vi "in_1d interp.vi"(7 "method":i32(ring) items=["nearest", "linear", "spline", "cubic Hermite", "Lagrange"], 9 "xi":dbl[](array[numeric]), 10 "Y":dbl[](array[numeric]), 11 "X":dbl[](array[numeric])) -> (0 "error":i32, 3 "yi":dbl[](array[numeric]))   [LabVIEW 2011, in "NI_Gmath.lvlib"]
uses:
  NI_Gmath.lvlib
  NI_AALPro.lvlib
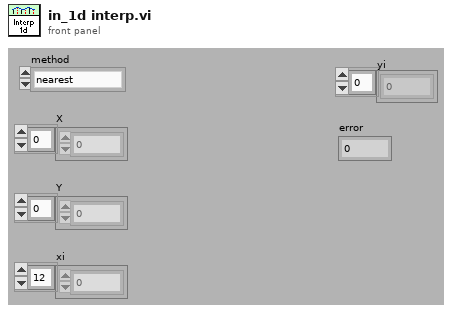
[diagram p1: front panel]
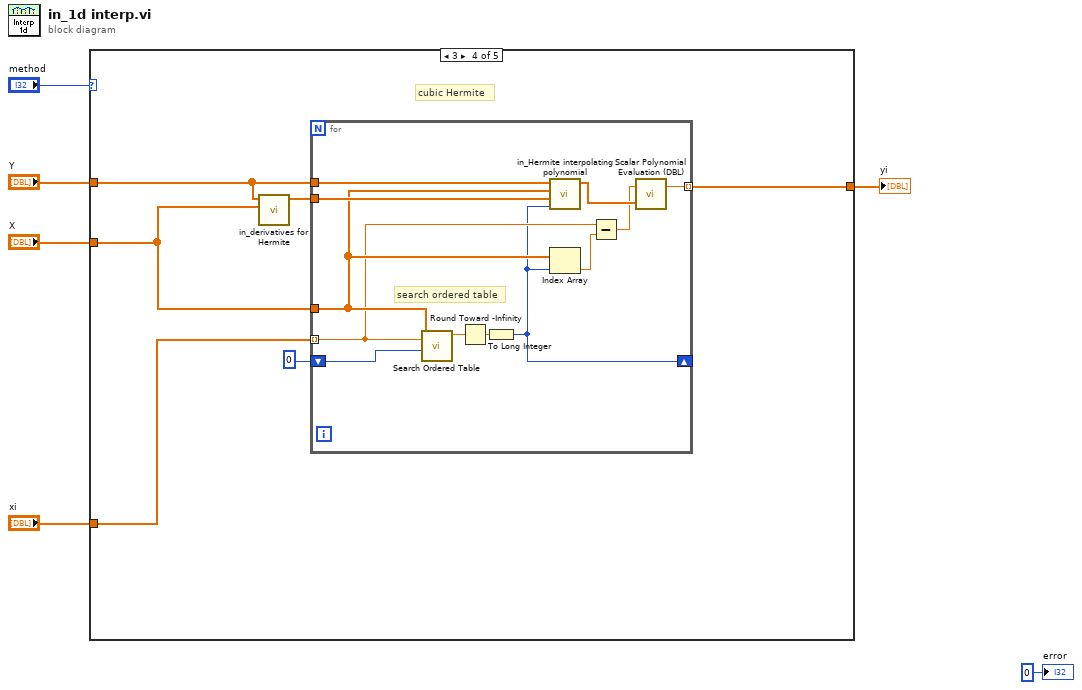
[diagram p0: block diagram]
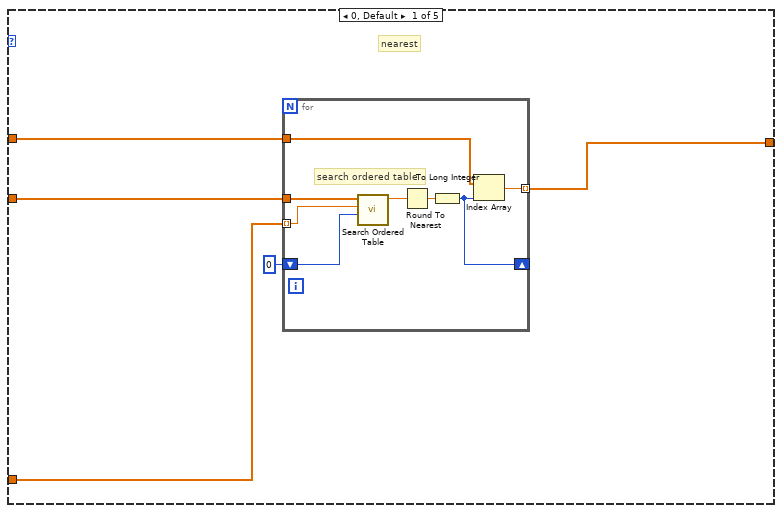
[diagram p2: hidden frame]
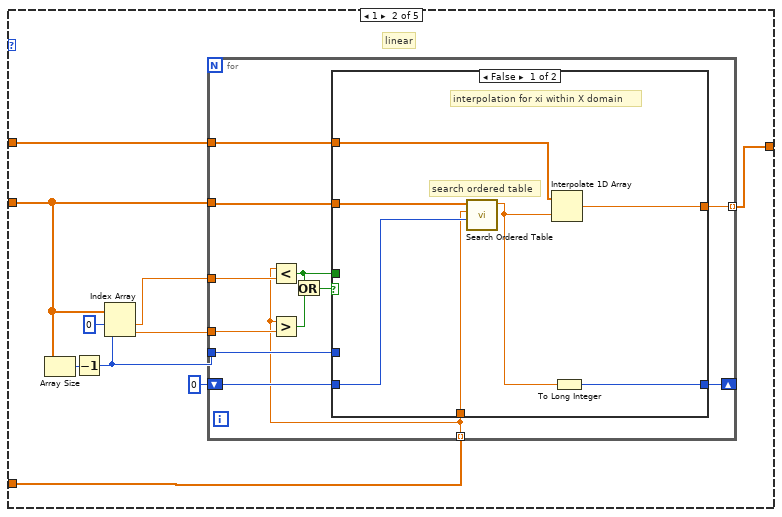
[diagram p3: hidden frame]
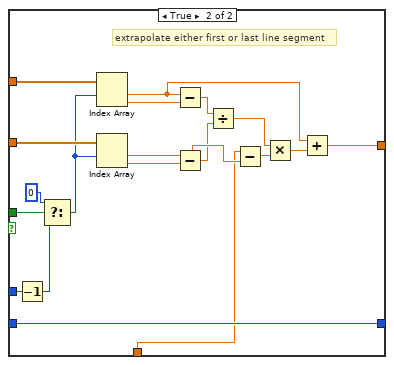
[diagram p4: hidden frame]
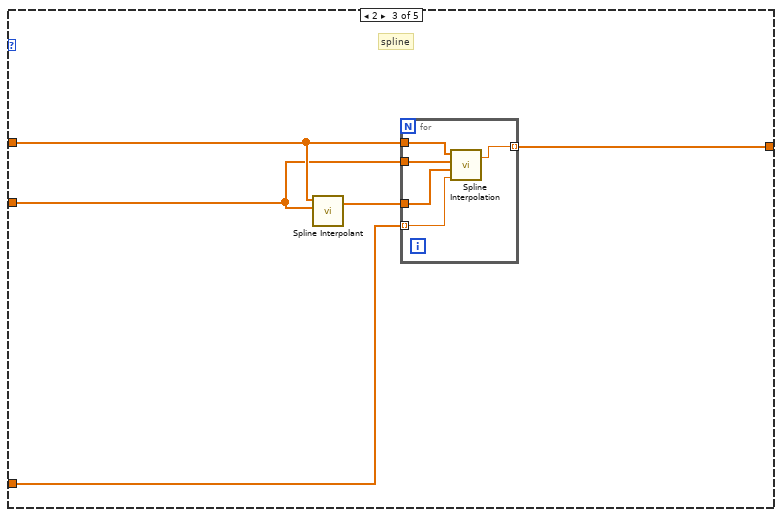
[diagram p5: hidden frame]
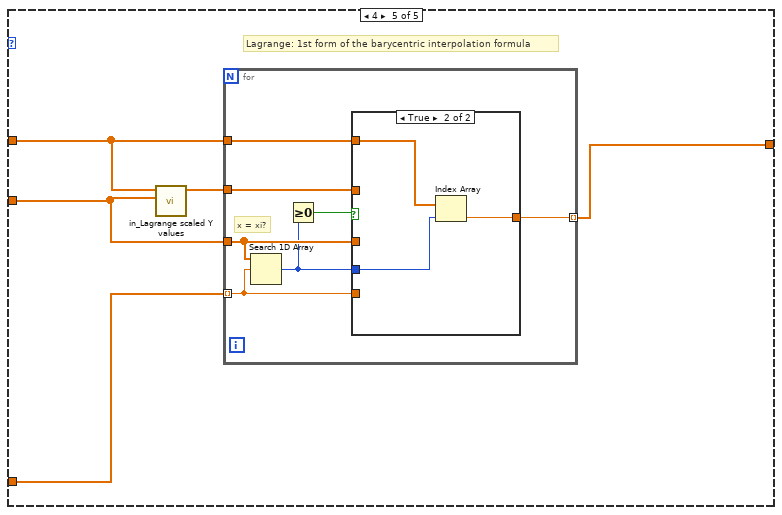
[diagram p6: hidden frame]
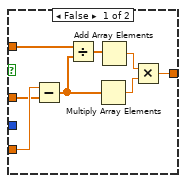
[diagram p7: hidden frame]
diagram:
  n1 = case shown="3" "method" {
    tunnel: "Y" -> [w7 w27 w72 w80 w96]
    tunnel: "X" -> [w9 w24 w71 w79 w99]
    tunnel: "xi" -> [w11 w21 w70 w83 w100]
    tunnel: [w10 w20 w68 w81 w97] -> w3
    frame 0, Default {
      # "nearest"
      n2 = for {
        tunnel: w9 -> [w16]
        tunnel: w11 -> [w15] mode=indexing
        tunnel: w7 -> [w18]
        tunnel: [w17] -> w10 mode=indexing
        shift-right: [w12] -> _
        shift-left: 0 -> [w14]
        # "search ordered table"
        n3 = call "Search Ordered Table.vi"("starting index"=w14, "x value"=w15, "ordered x array"=w16) -> ("fractional index"=w13:dbl)  [unwired: 8 in]
        n4 = Round To Nearest(number=w13) -> (nearest integer value=w19:dbl)
        n5 = To Long Integer(number=w19) -> (32bit integer=w12:i32)
        n6 = Index Array(array=w18, index=w12) -> (element=w17:dbl)
      }
    }
    frame 1 {
      # "linear"
      n7 = Array Size(array=w24) -> (size(s)=w25:i32)
      n8 = Decrement(x=w25) -> (x-1=w23:i32)
      n9 = Index Array(array=w24, index #1=0 ("index"), index #2=w23) -> (element #1=w28:dbl, element #2=w29:dbl)
      n10 = for {
        tunnel: w24 -> [w41]
        tunnel: w27 -> [w40]
        tunnel: [w39] -> w20 mode=indexing
        tunnel: w29 -> [w37]
        tunnel: w28 -> [w38]
        tunnel: w23 -> [w33]
        shift-right: [w31] -> _
        shift-left: 0 ("index") -> [w32]
        tunnel: w21 -> [w30] mode=indexing
        n11 = Less?(x=w30, y=w38) -> (x < y?=w35:bool)
        n12 = Greater?(x=w30, y=w37) -> (0:w34:bool)
        n13 = Or(x=w35, y=w34) -> (x .or. y?=w36:bool)
        n14 = case shown="False" w36 {
          tunnel: w41 -> [w46 w67]
          tunnel: w40 -> [w48 w66]
          tunnel: [w47 w65] -> w39
          tunnel: w35 -> [_ w53]
          tunnel: w33 -> [_ w64]
          tunnel: w32 -> [w45 w50]
          tunnel: [w42 w50] -> w31
          tunnel: w30 -> [w44 w49]
          frame False {
            # "search ordered table"
            # "interpolation for xi within X domain"
            n15 = call "Search Ordered Table.vi"("starting index"=w45, "x value"=w44, "ordered x array"=w46) -> ("fractional index"=w43:dbl)  [unwired: 8 in]
            n16 = Interpolate 1D Array(1:w43, 2:w48) -> (0:w47:dbl)
            n17 = To Long Integer(number=w43) -> (32bit integer=w42:i32)
          }
          frame True {
            # "extrapolate either first or last line segment"
            n18 = Decrement(x=w64) -> (x-1=w54:i32)
            n19 = Select(t=0, s=w53, f=w54) -> (s? t:f=w51:i32)
            n20 = Index Array(array=w66, index #1=w51) -> (element #1=w61:dbl, element #2=w63:dbl)  [unwired: 1 in]
            n21 = Index Array(array=w67, index #1=w51) -> (element #1=w60:dbl, element #2=w62:dbl)  [unwired: 1 in]
            n22 = Subtract(x=w61, y=w63) -> (x-y=w59:dbl)
            n23 = Subtract(x=w60, y=w62) -> (x-y=w58:dbl)
            n24 = Divide(x=w59, y=w58) -> (x/y=w56:dbl)
            n25 = Subtract(x=w49, y=w60) -> (x-y=w57:dbl)
            n26 = Multiply(x=w56, y=w57) -> (x*y=w55:dbl)
            n27 = Add(x=w61, y=w55) -> (x+y=w65:dbl)
          }
        }
      }
    }
    frame 2 {
      # "spline"
      n28 = call "Spline Interpolant.vi"("X"=w71, "Y"=w72) -> ("Interpolant"=w69:dbl[])  [unwired: 2 in, 1 out]
      n29 = for {
        tunnel: w72 -> [w77]
        tunnel: w71 -> [w76]
        tunnel: w70 -> [w75] mode=indexing
        tunnel: w69 -> [w74]
        tunnel: [w73] -> w68 mode=indexing
        n30 = call "Spline Interpolation.vi"("x value"=w75, "Interpolant"=w74, "X"=w76, "Y"=w77) -> ("interpolation value"=w73:dbl)  [unwired: 1 out]
      }
    }
    frame 3 {
      # "cubic Hermite"
      n31 = call "in_derivatives for Hermite.vi"("Y[0..N]"=w80, "X[0..N]"=w79) -> ("Y deriv[0..N]"=w82:dbl[])  [unwired: 8 in]
      n32 = for {
        tunnel: w79 -> [w90]
        tunnel: w83 -> [w86] mode=indexing
        tunnel: w80 -> [w95]
        tunnel: w82 -> [w91]
        tunnel: [w92] -> w81 mode=indexing
        shift-right: [w84] -> _
        shift-left: 0 -> [w85]
        # "search ordered table"
        n33 = call "Search Ordered Table.vi"("starting index"=w85, "x value"=w86, "ordered x array"=w90) -> ("fractional index"=w94:dbl)  [unwired: 8 in]
        n34 = Round Toward -Infinity(1:w94) -> (0:w89:dbl)
        n35 = To Long Integer(number=w89) -> (32bit integer=w84:i32)
        n36 = call "in_Hermite interpolating polynomial.vi"("index i"=w84, "Y deriv[0..N]"=w91, "X[0..N]"=w90, "Y[0..N]"=w95) -> ("Hermite polynomial"=w93:dbl[])  [unwired: 7 in]
        n37 = Index Array(array=w90, index=w84) -> (element=w87:dbl)
        n38 = Subtract(x=w86, y=w87) -> (x-y=w88:dbl)
        n39 = call "Scalar Polynomial Evaluation (DBL).vi"("P(x)"=w93, "a"=w88) -> ("P(a)"=w92:dbl)  [unwired: 1 out]
      }
    }
    frame 4 {
      # "Lagrange: 1st form of the barycentric interpolation formula"
      n40 = call "in_Lagrange scaled Y values.vi"("X[0..N]"=w99, "Y[0..N]"=w96) -> ("scaled Y"=w98:dbl[])  [unwired: 9 in]
      n41 = for {
        tunnel: w99 -> [w103]
        tunnel: w100 -> [w102] mode=indexing
        tunnel: w98 -> [w107]
        tunnel: [w106] -> w97 mode=indexing
        tunnel: w96 -> [w104]
        # "x = xi?"
        n42 = Search 1D Array(1D array=w103, element=w102) -> (index of element=w101:i32)  [unwired: 1 in]
        n43 = Greater Or Equal To 0?(x=w101) -> (x >= 0?=w105:bool)
        n44 = case shown="True" w105 {
          tunnel: w102 -> [w115 _]
          tunnel: w103 -> [w114 _]
          tunnel: w107 -> [w113 _]
          tunnel: [w109 w116] -> w106
          tunnel: w104 -> [_ w118]
          tunnel: w101 -> [_ w117]
          frame False {
            n45 = Subtract(x=w115, y=w114) -> (x-y=w108:dbl[])
            n46 = Divide(x=w113, y=w108) -> (x/y=w111:dbl[])
            n47 = Multiply Array Elements(1:w108) -> (0:w112:dbl)
            n48 = Add Array Elements(numeric array=w111) -> (sum=w110:dbl)
            n49 = Multiply(x=w110, y=w112) -> (x*y=w109:dbl)
          }
          frame True {
            n50 = Index Array(array=w118, index=w117) -> (element=w116:dbl)
          }
        }
      }
    }
  }
  "yi" <- w3
  "error" <- 0 ("error")
